vi "Main.vi"() -> ()   [LabVIEW 2021]
doc: "This template is for the Queued Message Handler design pattern.\n\nThe Event Handling Loop generates messages based on user interface actions.\n\nThe Message Handling Loop processes messages generated by the Event Handling Loop, or by other messages. The messages are string values, so new messages can be added easily to the Message Cases case structure in the Message Handling Loop. Each message cluster can also provide an optional value for Message Data, which is a variant that can be converted to whatever message-specific data is required."
uses:
  TypeDef/MotorControlCluster.ctl
  Muscle Actuator LabV Analog/Controls/Status Lights.ctl
  Muscle Actuator LabV Analog/Controls/DAQ Refnums.ctl
  support/Message Queue/Enqueue Message (Single).vi
  <vilib>/Utility/error.llb/Error Cluster From Error Code.vi
  <vilib>/ErrorRing/Error Ring.xnode
  support/Message Queue/Message Queue.lvlib
  support/User Event - Stop/User Event - Stop.lvlib
panel:
  out "Motor Control Cluster":T1
  out "Pressure":dbl format="%0.2f"
  in  "Speed":dbl(knob) min=0.0 max=5.0 scale=0.0..5.0
  in  "Simulate":bool
  out "Status":string
  in  "Exit":bool
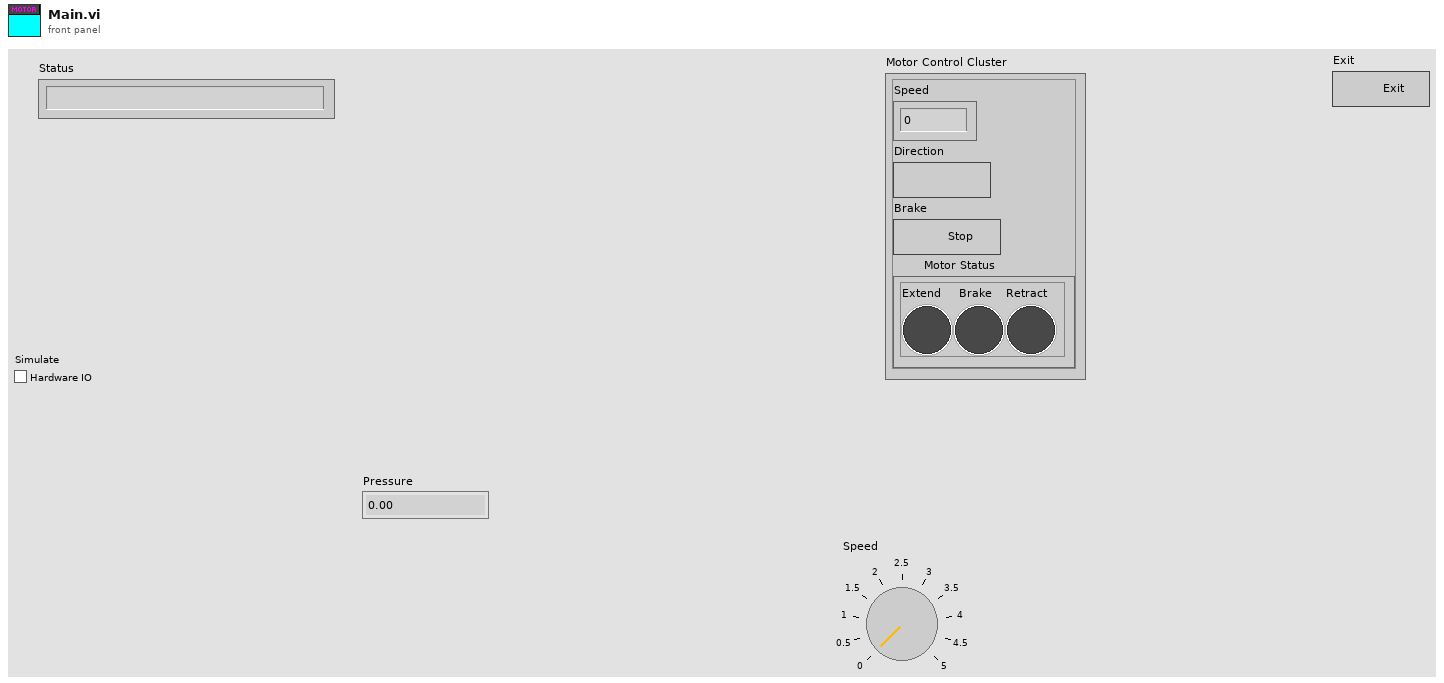
[diagram p1: front panel]
types:
  T1 = typedef "MotorControlCluster.ctl" = cluster{"Speed":dbl, "Direction":bool, "Brake":bool, "Motor Status":T2}
  T2 = typedef "Status Lights.ctl" = cluster{"Extend":bool, "Brake":bool, "Retract":bool}
  T3 = typedef "DAQ Refnums.ctl" = cluster{"Direction Ref":refnum<k21>, "Brake Ref":refnum<k21>, "Speed Ref":refnum<k21>, "Pressure Ref":refnum<k21>}
  T4 = typedef "Message Queue.lvlib/All Message Queues.ctl" = cluster{"UI":refnum<queue>}
  T5 = typedef "eventvkey.ctl" = enum16{"ASCII", "Enter", "Return", "Shift", "Ctrl", "Alt", "Cmd", "Opt", "Caps", "NumLock", "Clear", "Break", "Up", "Down", "Left", "Right", "Insert", "Delete", "Home", "End", "PageUp", "PageDown", "Escape", "Help", "Pause", "ScrollLock", "F1", "F2", "F3", "F4", "F5", "F6", "F7", "F8", "F9", "F10", "F11", "F12", "F13", "F14", "F15", "F16", "F17", "F18", "F19", "F20", "F21", "F22", "F23", "F24", "Play", "VolumeUp", "VolumeDown", "Mute", "Two Byte Char"}
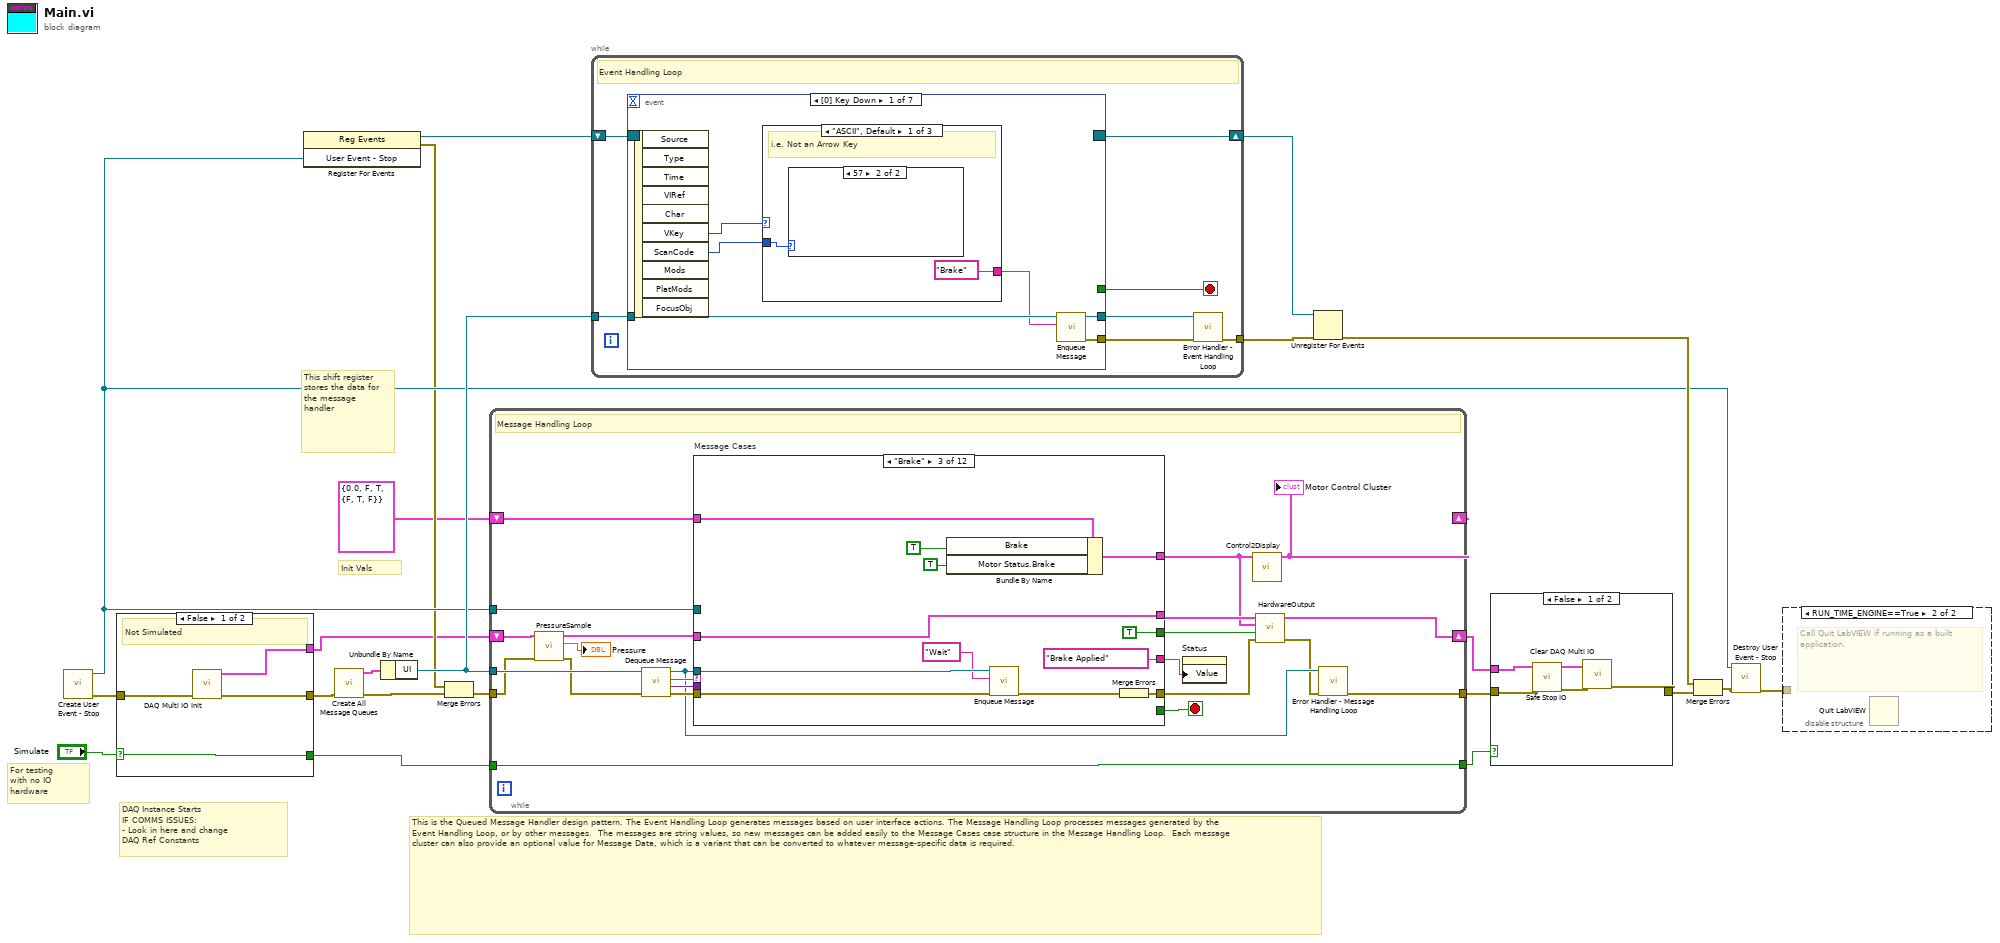
[diagram p0: block diagram]
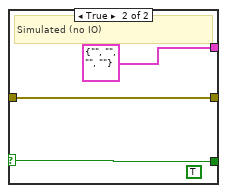
[diagram p3: hidden frame]
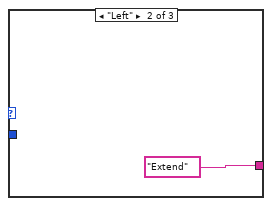
[diagram p6: hidden frame]
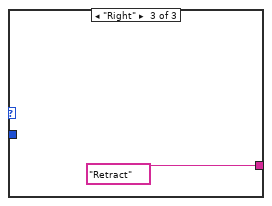
[diagram p7: hidden frame]
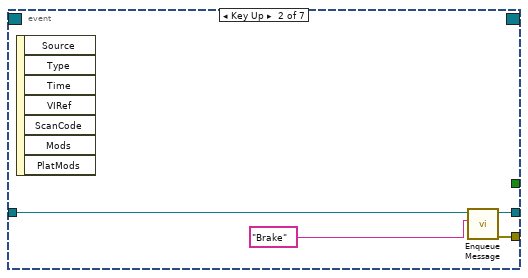
[diagram p8: hidden frame]
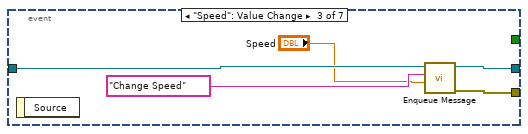
[diagram p9: hidden frame]
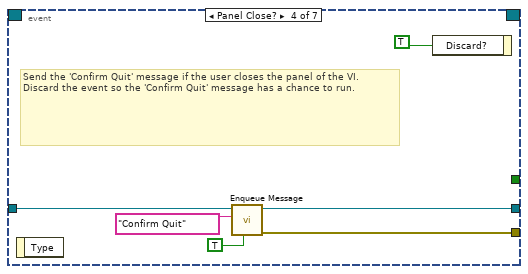
[diagram p10: hidden frame]
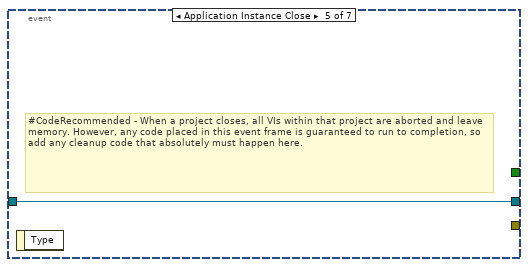
[diagram p11: hidden frame]
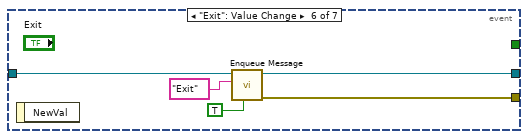
[diagram p12: hidden frame]
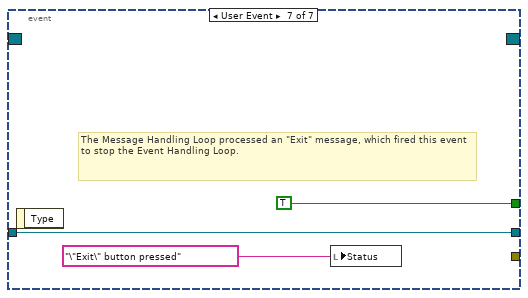
[diagram p13: hidden frame]
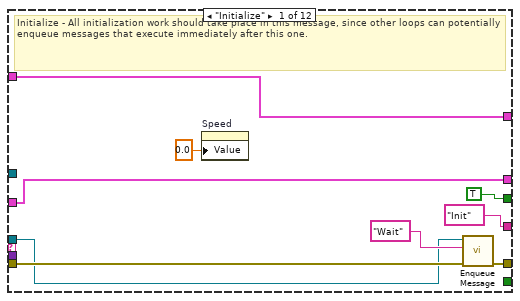
[diagram p14: hidden frame]
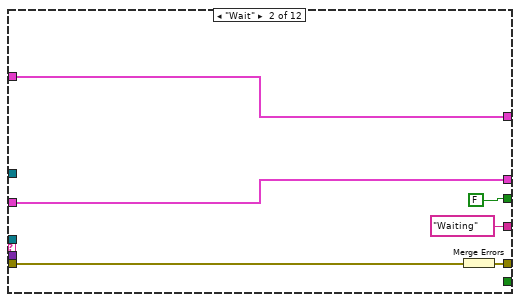
[diagram p15: hidden frame]
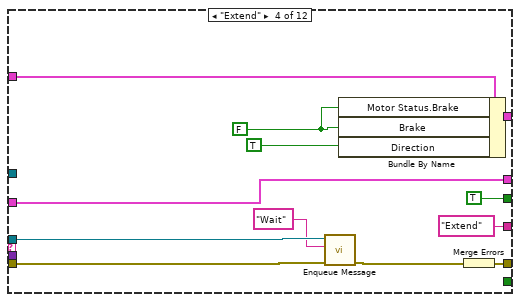
[diagram p16: hidden frame]
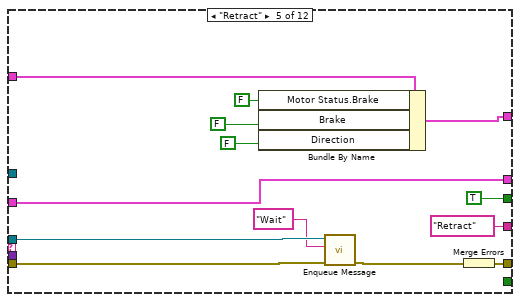
[diagram p17: hidden frame]
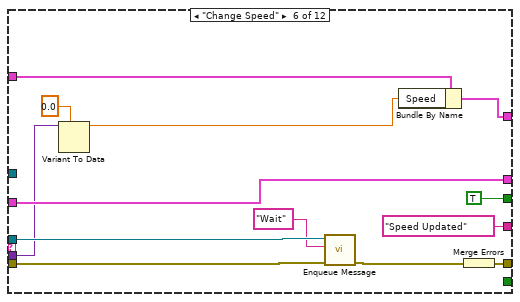
[diagram p18: hidden frame]
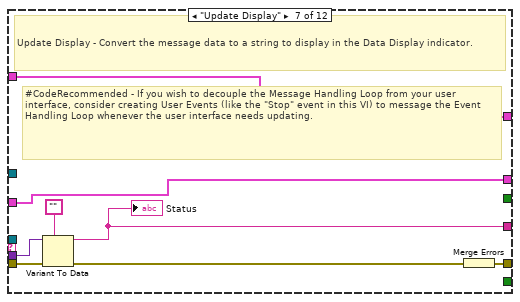
[diagram p19: hidden frame]
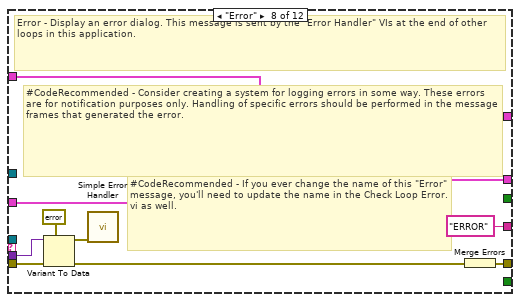
[diagram p20: hidden frame]
diagram:
  # "Init Vals"
  # "For testing \nwith no IO\nhardware"
  # "DAQ Instance Starts\nIF COMMS ISSUES:\n- Look in here and change\nDAQ Ref Constants"
  # "This is the Queued Message Handler design pattern. The Event Handling Loop generates messages based on user interface actions. The Message Handling Loop processes messages generated by the Event Handling Loop, or by other messages.  The messages are string values, so new messages can be added easily to the Message Cases case structure in the Message Handling Loop.  Each message cluster can also provide an optional value for Message Data, which is a variant that can be converted to whatever message-specific data is required."
  # "This shift register stores the data for the message handler"
  n1 = call "Create User Event - Stop.vi"() -> ("error out"=w10:errorcluster, "User Event - Stop"=w13:refnum<user-event>)  [unwired: 10 in]
  n2 = case shown="False" "Simulate" {
    selector: "Simulate" -> [w23 w27]
    tunnel: w10 -> [w26 w28]
    tunnel: [w25 w28] -> w9
    tunnel: [w24 T3 {"Direction Ref"="", "Brake Ref"="", "Speed Ref"="", "Pressure Ref"=""} ("DAQ Ref Cluster")] -> w8
    tunnel: [w23 w27] -> w2
    frame False {
      # "Not Simulated"
      n3 = call "DAQ Multi IO Init.vi"("error in"=w26) -> ("error out"=w25:errorcluster, "DAQ Ref Cluster"=w24:T3)  [unwired: 9 in]
    }
    frame True {
      (unwired) TRUE ("Visible")
      # "Simulated (no IO)"
    }
  }
  n4 = register-events(w13) -> (reference out=w14:refnum<event-registration>, error out=w11:errorcluster)  [unwired: 2 in]
  n5 = call "Create All Message Queues.vi"("error in (no error)"=w9) -> ("error out"=w22:errorcluster, "Message Queues out"=w21:T4)  [unwired: 9 in]
  n6 = Unbundle By Name(w21) -> ("UI"=w20:refnum<queue>)
  n7 = Merge Errors(w11, w22) -> (w12:errorcluster)
  n8 = while {
    tunnel: w20 -> [w46]
    shift-right: [w30] -> _
    shift-left: T1 {"Speed"=0.0, "Direction"=FALSE, "Brake"=TRUE, "Motor Status"={"Extend"=FALSE, "Brake"=TRUE, "Retract"=FALSE}} ("Motor Control Cluster") -> [w52]
    tunnel: w13 -> [w50]
    tunnel: w12 -> [w43]
    tunnel: [w44] -> w5
    shift-right: [w37] -> w4
    shift-left: w8 -> [w42]
    tunnel: [w32] -> w1
    tunnel: w2 -> [w32]
    stop <- w51 stop-if-true
    # "Message Handling Loop"
    n9 = call "PressureSample.vi"("error in (no error)"=w43, "DAQREFS"=w42) -> ("error out"=w38:errorcluster, "Voltage"=→"Pressure":dbl, "DAQREFs"=w39:T3)  [unwired: 7 in]
    n10 = call "Dequeue Message.vi"("error in (no error)"=w38, "Message Queue"=w46) -> ("error out"=w49:errorcluster, "Message Data"=w47:variant, "Message"=w48:string, "dup Message Queue"=w45:refnum<queue>)  [unwired: 6 in]
    n11 = case "Message Cases" shown="\"Brake\"" w48 {
      selector: w48 -> [_ _ _ _ _ _ _ _ _ _ _ w164]
      tunnel: w45 -> [w58 _ w72 w85 w97 w111 _ _ w139 _ w161 _]
      tunnel: w49 -> [w60 w64 w71 w84 w96 w110 w123 w134 w143 w148 w154 _]
      tunnel: [w61 w66 w79 w91 w104 w117 w124 w128 w141 w146 w157 w165] -> w35
      tunnel: w52 -> [w55 w67 w74 w86 w99 w112 w125 w133 w142 w147 w160 w166]
      tunnel: [w55 w67 w75 w87 w100 w113 w125 w133 w142 w147 w160 w166] -> w31
      tunnel: [_ _ _ _ _ _ _ _ _ _ TRUE _] -> w51
      tunnel: w47 -> [_ _ _ _ _ w107 w122 w132 _ _ w151 _]
      tunnel: w50 -> [_ _ _ _ _ _ _ _ _ _ w156 _]
      tunnel: w39 -> [w54 w65 w78 w90 w103 w116 w119 w126 w135 w144 w149 w162]
      tunnel: ["Init" ("Initial Message") "Waiting" ("Initial Message") "Brake Applied" ("Initial Message") "Extend" ("Initial Message") "Retract" ("Initial Message") "Speed Updated" ("Initial Message") w118 "ERROR" ("Initial Message") "Quitting" ("Initial Message") "Copy" ("Initial Message") "Exit" ("Initial Message") "ERROR: INVALID MESSAGE" ("Initial Message")] -> w40
      tunnel: [w54 w65 w78 w90 w103 w116 w119 w126 w135 w144 w149 w162] -> w36
      tunnel: [TRUE FALSE TRUE TRUE TRUE TRUE _ _ _ _ _ _] -> w33
      frame "Initialize" {
        # "Initialize - All initialization work should take place in this message, since other loops can potentially enqueue messages that execute immediately after this one."
        n12 = property on="Speed" class="Knob (strict)"("Value"=0.0 ("Speed")) -> ()  [unwired: 2 in, 2 out]
        n13 = call-poly "Enqueue Message.vi"("error in (no error)"=w60, "Message"="Wait", "Message Queue"=w58) -> ("error out"=w61:errorcluster)  [unwired: 7 in, 1 out]
      }
      frame "Wait" {
        n14 = Merge Errors(w64) -> (w66:errorcluster)
      }
      frame "Brake" {
        n15 = Bundle By Name(cluster=w74, "Brake"=TRUE, "Motor Status.Brake"=TRUE) -> (w75:T1)
        n16 = call-poly "Enqueue Message.vi"("error in (no error)"=w71, "Message"="Wait", "Message Queue"=w72) -> ("error out"=w70:errorcluster)  [unwired: 7 in, 1 out]
        n17 = Merge Errors(w70) -> (w79:errorcluster)
      }
      frame "Extend" {
        w80 = FALSE ("Brake")
        n18 = call-poly "Enqueue Message.vi"("error in (no error)"=w84, "Message"="Wait", "Message Queue"=w85) -> ("error out"=w83:errorcluster)  [unwired: 7 in, 1 out]
        n19 = Bundle By Name(cluster=w86, "Motor Status.Brake"=w80, "Brake"=w80, "Direction"=TRUE) -> (w87:T1)
        n20 = Merge Errors(w83) -> (w91:errorcluster)
      }
      frame "Retract" {
        n21 = Bundle By Name(cluster=w99, "Motor Status.Brake"=FALSE, "Brake"=FALSE, "Direction"=FALSE) -> (w100:T1)
        n22 = call-poly "Enqueue Message.vi"("error in (no error)"=w96, "Message"="Wait", "Message Queue"=w97) -> ("error out"=w95:errorcluster)  [unwired: 7 in, 1 out]
        n23 = Merge Errors(w95) -> (w104:errorcluster)
      }
      frame "Change Speed" {
        n24 = Variant To Data(type=0.0 ("Speed"), Variant=w107) -> (data=w105:dbl)  [unwired: 1 in, 1 out]
        n25 = call-poly "Enqueue Message.vi"("error in (no error)"=w110, "Message"="Wait", "Message Queue"=w111) -> ("error out"=w109:errorcluster)  [unwired: 7 in, 1 out]
        n26 = Bundle By Name(cluster=w112, "Speed"=w105) -> (w113:T1)
        n27 = Merge Errors(w109) -> (w117:errorcluster)
      }
      frame "Update Display" {
        # "#CodeRecommended - If you wish to decouple the Message Handling Loop from your user interface, consider creating User Events (like the \"Stop\" event in this VI) to message the Event Handling Loop whenever the user interface needs updating."
        # "Update Display - Convert the message data to a string to display in the Data Display indicator."
        n28 = Variant To Data(error in=w123, type="", Variant=w122) -> (data=w118:string, error out=w120:errorcluster)
        "Status" <- w118
        n29 = Merge Errors(w120) -> (w124:errorcluster)
      }
      frame "Error" {
        # "#CodeRecommended - If you ever change the name of this \"Error\" message, you'll need to update the name in the Check Loop Error.vi as well."
        # "#CodeRecommended - Consider creating a system for logging errors in some way. These errors are for notification purposes only. Handling of specific errors should be performed in the message frames that generated the error."
        # "Error - Display an error dialog. This message is sent by the \"Error Handler\" VIs at the end of other loops in this application."
        n30 = Variant To Data(error in=w134, type=errorcluster {"status"=FALSE, "code"=0, "source"=""} ("error constant"), Variant=w132) -> (data=w130:errorcluster, error out=w129:errorcluster)
        n31 = call <vilib>:"Simple Error Handler.vi"("error in (no error)"=w130) -> ()  [unwired: 4 in, 5 out]
        n32 = Merge Errors(w129) -> (w128:errorcluster)
      }
      frame "Confirm Quit" {
        # "#CodeNeeded - If you want to provide an \"Are you sure\" dialog (or some other notification) before the application exits, place that code here. This message is typically sent from a Panel Close? event."
        # "Confirm Quit - Message that can confirm whether or not the user wants to exit the application."
        n33 = call-poly "Enqueue Message.vi"("Priority Message? (F)"=TRUE, "error in (no error)"=w143, "Message"="Exit", "Message Queue"=w139) -> ("error out"=w140:errorcluster)  [unwired: 6 in, 1 out]
        n34 = Merge Errors(w140) -> (w141:errorcluster)
      }
      frame "---Copy This Frame---" {
        # "Duplicate this frame when creating new messages.  Change this comment in the duplicated frame to describe this message."
        n35 = Merge Errors(w148) -> (w146:errorcluster)
      }
      frame "Exit" {
        # "Stop the VI"
        # "Release the message queue reference"
        # "#CodeNeeded - Add any required cleanup code here. Note that if 'Exit' was called as a result of an error, an error dialog will be displayed. Add any custom error handling for an 'Exit' condition here as well."
        # "Exit - Exit the application."
        n36 = Variant To Data(type=errorcluster {"status"=FALSE, "code"=0, "source"=""} ("error constant"), Variant=w151) -> (data=w152:errorcluster)  [unwired: 1 in, 1 out]
        n37 = call <vilib>:"Simple Error Handler.vi"("error in (no error)"=w152) -> ()  [unwired: 4 in, 5 out]
        n38 = call "Fire User Event - Stop.vi"("User Event - Stop"=w156) -> ("error out"=w155:errorcluster)  [unwired: 10 in]
        n39 = Release Queue(queue=w161, error in (no error)=w154) -> (error out=w158:errorcluster)  [unwired: 1 in, 2 out]
        n40 = Merge Errors(w155, w158) -> (w157:errorcluster)
      }
      frame Default {
        # "'Default' case only runs if there is a message that isn't defined in any of the other cases.  Output a programming error."
        n41 = xnode "Error Ring"("parameter 0"=w164) -> ("error out"=w165:errorcluster)
      }
    }
    n42 = property on="Status" class="Str"("Value"=w40) -> ()  [unwired: 2 in, 2 out]
    n43 = call "Control2Display.vi"("Motor Control Cluster"=w31) -> ("Motor Control Cluster"=w30:T1)  [unwired: 10 in]
    "Motor Control Cluster" <- w30
    n44 = call "HardwareOutput.vi"("error in"=w35, "Update Outputs"=w33, "Motor Control Cluster"=w31, "DAQREFs in"=w36) -> ("error out"=w34:errorcluster, "DAQREFs out"=w37:T3)  [unwired: 6 in]
    n45 = call "Error Handler - Message Handling Loop.vi"("error in (no error)"=w34, "Message Queue"=w45) -> ("dup error in"=w44:errorcluster)  [unwired: 8 in, 1 out]
  }
  n46 = while {
    tunnel: w20 -> [w180]
    shift-right: [w178] -> w17
    shift-left: w14 -> [w179]
    tunnel: [w174] -> w15
    stop <- w176 stop-if-true
    # "Event Handling Loop"
    n47 = event shown="[0] Key Down" {
      selector: w179 -> [_ _ _ _ _ _ _]
      dyn-events: [_ _ _ _ _ _ _] -> w178
      timeout: _ -> [_ _ _ _ _ _ _]
      tunnel: [_ _ _ _ _ _ TRUE ("Discard?")] -> w176
      tunnel: w180 -> [w186 w194 w199 w205 w206 w211 w214]
      tunnel: [w184 w192 w196 w204 _ w210 _] -> w177
      tunnel: [w185 w193 w198 w203 w206 w209 w214] -> w175
      event Key Down {
        n48 = event-data() -> ("VKey"=w183:T5, "ScanCode"=w182:i16)  [unwired: 1 in, 8 out]
        n49 = case shown="\"ASCII\", Default" w183 {
          tunnel: w182 -> [w188 _ _]
          tunnel: ["Brake" ("Message") "Extend" ("Message") "Retract" ("Message")] -> w181
          frame "ASCII", Default {
            # "i.e. Not an Arrow Key"
            n50 = case shown="57" w188 {
              frame Default {
              }
              frame 57 {
              }
            }
          }
          frame "Left" {
          }
          frame "Right" {
          }
        }
        n51 = call-poly "Enqueue Message.vi"("Message"=w181, "Message Queue"=w186) -> ("error out"=w184:errorcluster, "dup Message Queue"=w185:refnum<queue>)  [unwired: 8 in]
      }
      event Key Up {
        n52 = event-data() -> ()  [unwired: 1 in, 7 out]
        n53 = call-poly "Enqueue Message.vi"("Message"="Brake", "Message Queue"=w194) -> ("error out"=w192:errorcluster, "dup Message Queue"=w193:refnum<queue>)  [unwired: 8 in]
      }
      event "Speed": Value Change {
        n54 = event-data() -> ()  [unwired: 1 in, 1 out]
        n55 = call-poly "Enqueue Message.vi"("Message Data"="Speed", "Message"="Change Speed", "Message Queue"=w199) -> ("error out"=w196:errorcluster, "dup Message Queue"=w198:refnum<queue>)  [unwired: 7 in]
      }
      event Panel Close? {
        # "Send the 'Confirm Quit' message if the user closes the panel of the VI. Discard the event so the 'Confirm Quit' message has a chance to run."
        n56 = event-data() -> ()  [unwired: 1 in, 1 out]
        n57 = call-poly "Enqueue Message.vi"("Priority Message? (F)"=TRUE, "Message"="Confirm Quit", "Message Queue"=w205) -> ("error out"=w204:errorcluster, "dup Message Queue"=w203:refnum<queue>)  [unwired: 7 in]
        n58 = event-data("Discard?"=TRUE) -> ()  [unwired: 1 in, 1 out]
      }
      event Application Instance Close {
        # "#CodeRecommended - When a project closes, all VIs within that project are aborted and leave memory. However, any code placed in this event frame is guaranteed to run to completion, so add any cleanup code that absolutely must happen here."
        n59 = event-data() -> ()  [unwired: 1 in, 1 out]
      }
      event "Exit": Value Change {
        n60 = event-data() -> ()  [unwired: 1 in, 1 out]
        n61 = call-poly "Enqueue Message.vi"("Priority Message? (F)"=TRUE, "Message"="Exit", "Message Queue"=w211) -> ("error out"=w210:errorcluster, "dup Message Queue"=w209:refnum<queue>)  [unwired: 7 in]
      }
      event User Event {
        # "The Message Handling Loop processed an \"Exit\" message, which fired this event to stop the Event Handling Loop."
        n62 = event-data() -> ()  [unwired: 1 in, 1 out]
        n63 = local write "Status"("\"Exit\" button pressed" ("VI Stopped")) -> ()
      }
    }
    n64 = call "Error Handler - Event Handling Loop.vi"("error in (no error)"=w177, "Message Queue"=w175) -> ("dup error in"=w174:errorcluster)  [unwired: 8 in, 1 out]
  }
  n65 = Unregister For Events(event registration refnum=w17, error in=w15) -> (error out=w18:errorcluster)
  n66 = case shown="False" w1 {
    tunnel: [w219 w220] -> w3
    tunnel: w4 -> [w218 _]
    tunnel: w5 -> [w217 w220]
    frame False {
      n67 = call "Safe Stop IO.vi"("error in"=w217, "DAQ Ref Cluster"=w218) -> ("error out"=w215:errorcluster, "DAQ Ref Cluster Out"=w216:T3)  [unwired: 8 in]
      n68 = call "Clear DAQ Multi IO.vi"("error in"=w215, "DAQ Ref"=w216) -> ("error out"=w219:errorcluster)  [unwired: 9 in]
    }
    frame True {
    }
  }
  n69 = Merge Errors(w18, w3) -> (w19:errorcluster)
  n70 = call "Destroy User Event - Stop.vi"("error in (no error)"=w19, "User Event - Stop"=w13) -> ("error out"=w16:errorcluster)  [unwired: 9 in]
  n71 = disable-structure shown="RUN_TIME_ENGINE==True" {
    disable-tunnel: w16 -> [_ _]
    frame condition #0 (active) {
    }
    frame condition #1 {
      # "Call Quit LabVIEW if running as a built application."
      n72 = Quit LabVIEW() -> ()  [unwired: 1 in]
    }
  }
